vi "DC_CNTRL_initialise.vi"(7 "Check status?":bool, 8 "error in (no error)":errorcluster, 10 "Box Number":i32, 11 "Device Index":u32) -> (0 "error out":errorcluster, 1 "Device Information":T1 {"Type" items=["FT232B-FT245B", "FT8U232AM-FT8U245AM", "FT8U100AX", "UNKNOWN", "FT2232", "FT232R-FT245R", "FT2232H", "FT4232H", "FT232H"]}, 3 "Handle out":u64)   [LabVIEW 2019]
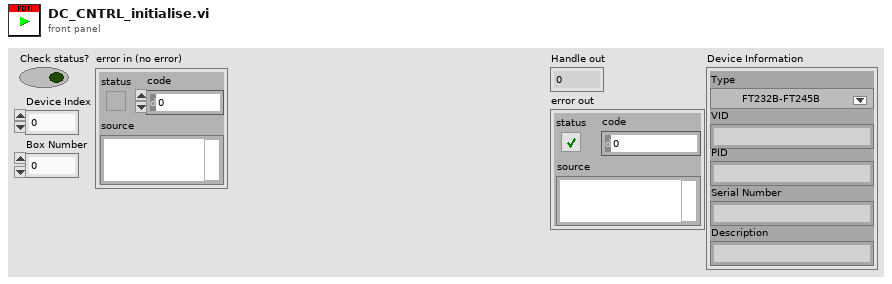
[diagram p1: front panel]
types:
  T1 = cluster{"Type":u32, "VID":string, "PID":string, "Serial Number":string, "Description":string}
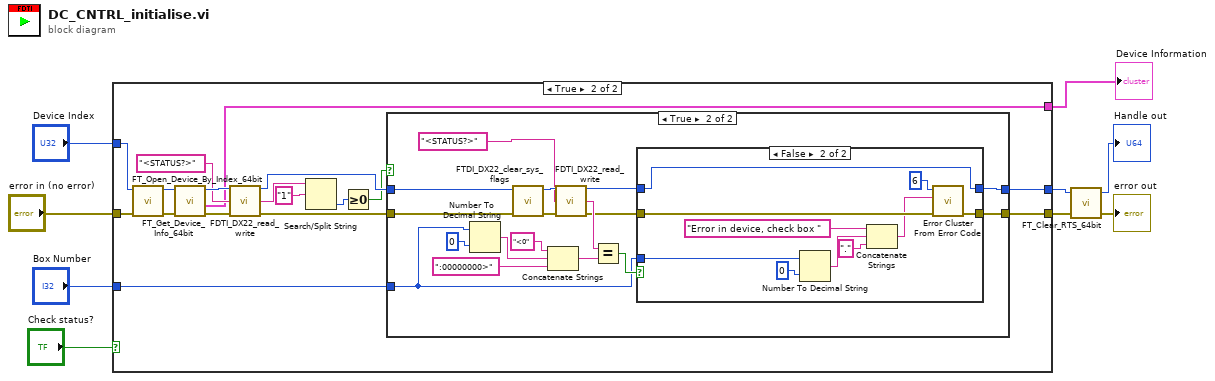
[diagram p0: block diagram]
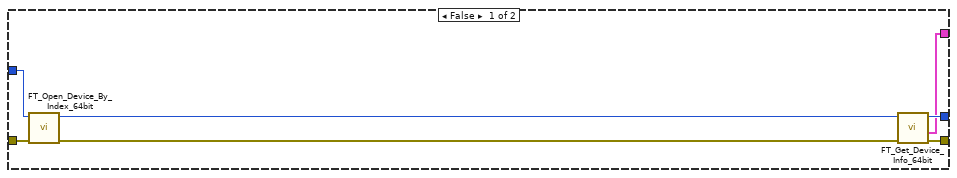
[diagram p2: hidden frame]
diagram:
  n1 = case shown="True" "Check status?" {
    tunnel: "Device Index" -> [w16 w33]
    tunnel: "error in (no error)" -> [w15 w32]
    tunnel: "Box Number" -> [_ w20]
    tunnel: [w12 w19] -> w5
    tunnel: [w11 w18] -> w4
    tunnel: [w10 w17] -> w1
    frame False {
      n2 = call "FT_Open_Device_By_Index_64bit.vi"("error in (no error)"=w15, "Device Index"=w16) -> ("error out"=w13:errorcluster, "Handle"=w14:u64)  [unwired: 6 in, 1 out]
      n3 = call "FT_Get_Device_Info_64bit.vi"("error in (no error)"=w13, "Handle"=w14) -> ("error out"=w11:errorcluster, "Device Information"=w10:T1, "Handle out"=w12:u64)  [unwired: 6 in, 1 out]
    }
    frame True {
      n4 = call "FT_Open_Device_By_Index_64bit.vi"("error in (no error)"=w32, "Device Index"=w33) -> ("error out"=w30:errorcluster, "Handle"=w31:u64)  [unwired: 6 in, 1 out]
      n5 = call "FT_Get_Device_Info_64bit.vi"("error in (no error)"=w30, "Handle"=w31) -> ("error out"=w28:errorcluster, "Device Information"=w17:T1, "Handle out"=w29:u64)  [unwired: 6 in, 1 out]
      n6 = call "FDTI_DX22_read_write.vi"("Handle"=w29, "Write string"="<STATUS?>", "error in (no error)"=w28) -> ("Handle out"=w23:u64, "Read Data"=w26:string, "error out"=w21:errorcluster)  [unwired: 10 in]
      n7 = Search/Split String(string=w26, search string/char (-)="1") -> (offset of match=w24:i32)  [unwired: 1 in, 2 out]
      n8 = Greater Or Equal To 0?(x=w24) -> (x >= 0?=w22:bool)
      n9 = case shown="True" w22 {
        tunnel: w23 -> [w35 w52]
        tunnel: w21 -> [w34 w51]
        tunnel: w20 -> [_ w37]
        tunnel: [w35 w39] -> w19
        tunnel: [w34 w38] -> w18
        frame False {
        }
        frame True {
          n10 = Number To Decimal String(number=w37, width (-)=i16 0) -> (decimal integer string=w40:string)
          n11 = call "FTDI_DX22_clear_sys_flags.vi"("error in (no error)"=w51, "Handle"=w52) -> ("error out"=w49:errorcluster, "Handle out"=w50:u64)  [unwired: 8 in]
          n12 = Concatenate Strings("<0" ("string"), w40, ":00000000>" ("string")) -> (w44:string)
          n13 = call "FDTI_DX22_read_write.vi"("Handle"=w50, "Write string"="<STATUS?>", "error in (no error)"=w49) -> ("Handle out"=w42:u64, "Read Data"=w48:string, "error out"=w41:errorcluster)  [unwired: 10 in]
          n14 = Equal?(x=w48, y=w44) -> (x = y?=w43:bool)
          n15 = case shown="False" w43 {
            tunnel: w42 -> [w54 w62]
            tunnel: w41 -> [w53 w63]
            tunnel: [w54 w62] -> w39
            tunnel: [w53 w61] -> w38
            tunnel: w37 -> [_ w59]
            frame True {
            }
            frame False {
              n16 = Number To Decimal String(number=w59, width (-)=i16 0) -> (decimal integer string=w57:string)
              n17 = Concatenate Strings("Error in device, check box " ("error message (\"\")"), w57, "." ("string")) -> (w55:string)
              n18 = call <vilib>:"Error Cluster From Error Code.vi"("error in (no error)"=w63, "error message (\"\")"=w55, "error code (0)"=6) -> ("error out"=w61:errorcluster)  [unwired: 6 in]
            }
          }
        }
      }
    }
  }
  "Device Information" <- w1
  n19 = call "FT_Clear_RTS_64bit.vi"("error in (no error)"=w4, "Handle"=w5) -> ("error out"=→"error out":errorcluster, "Handle out"=→"Handle out":u64)  [unwired: 1 in, 1 out]
